vi "test_ReserveSessionForPinGroup_ReserveSuccessForPinsInGroup.vi"() -> (6 "pass":bool, 8 "result":string, 15 "error out":errorcluster)   [LabVIEW 2020]
uses:
  Runtime/MeasurementLink Pin Map Client/RPC Messages/ni_measurementlink_pinmap_v1_CreatePinMapFromXmlRequest.ctl
  Runtime/MeasurementLink Session Management Client/RPC Messages/ni_measurementlink_sessionmanagement_v1_ReserveSessionsRequest.ctl
  Runtime/MeasurementLink Session Management Client/RPC Messages/ni_measurementlink_PinMapContext.ctl
  Runtime/MeasurementLink Session Management Client/RPC Messages/ni_measurementlink_sessionmanagement_v1_ReserveAllRegisteredSessionsResponse.ctl
  3347d1b6-dca7-4e1a-9ca0-c9ec2f5aba95.vi
  ab61e54b-70f9-4719-86d2-c3025959eeb5.vi
  <vilib>/JDP Science/JSONtext/Variant to JSON Text.vi
  <vilib>/JDP Science/JSONtext/LVClass Serializer/JSONtext LVClass Serializer.lvclass
  Runtime/MeasurementLink Session Management Client/MeasurementLink Session Management Client.lvlib
  Runtime/MeasurementLink Pin Map Client/MeasurementLink Pin Map Client.lvlib
  Runtime/MeasurementLink Session Management Client/RPC Messages/ni_measurementlink_sessionmanagement_v1_ChannelMapping.ctl
  Runtime/MeasurementLink Session Management Client/RPC Messages/nidevice_grpc_Session.ctl
  Runtime/MeasurementLink Session Management Client/RPC Messages/ni_measurementlink_sessionmanagement_v1_SessionInformation.ctl
  Runtime/MeasurementLink Session Management Client/RPC Messages/ni_measurementlink_sessionmanagement_v1_MultiplexerSessionInformation.ctl
  Runtime/MeasurementLink Session Management Client/RPC Messages/ni_measurementlink_sessionmanagement_v1_ResolvedPinsOrRelays.ctl
  Runtime/MeasurementLink Session Management Client/RPC Messages/ni_measurementlink_sessionmanagement_v1_ReserveSessionsResponse_GroupMappingsEntry.ctl
  Runtime/MeasurementLink Session Management Client/RPC Messages/ni_measurementlink_sessionmanagement_v1_ReserveSessionsResponse.ctl
panel:
  # "Test assumes discovery service, pin map service, and session management service have already been started."
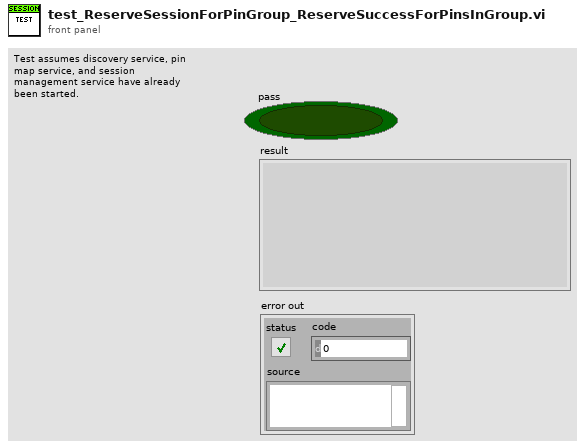
[diagram p1: front panel]
types:
  T1 = typedef "MeasurementLink Session Management Client.lvlib/ni_measurementlink_sessionmanagement_v1_ReserveSessionsResponse.ctl" = cluster{"sessions":T2[], "multiplexer_sessions":T5[], "group_mappings":T6[]}
  T2 = typedef "MeasurementLink Session Management Client.lvlib/ni_measurementlink_sessionmanagement_v1_SessionInformation.ctl" = cluster{"session":T3, "resource_name":string, "channel_list":string, "instrument_type_id":string, "session_exists":bool, "channel_mappings":T4[]}
  T3 = typedef "MeasurementLink Session Management Client.lvlib/nidevice_grpc_Session.ctl" = cluster{"name":string}
  T4 = typedef "MeasurementLink Session Management Client.lvlib/ni_measurementlink_sessionmanagement_v1_ChannelMapping.ctl" = cluster{"pin_or_relay_name":string, "site":i32, "channel":string, "multiplexer_resource_name":string, "multiplexer_route":string}
  T5 = typedef "MeasurementLink Session Management Client.lvlib/ni_measurementlink_sessionmanagement_v1_MultiplexerSessionInformation.ctl" = cluster{"session":T3, "resource_name":string, "multiplexer_type_id":string, "session_exists":bool}
  T6 = typedef "MeasurementLink Session Management Client.lvlib/ni_measurementlink_sessionmanagement_v1_ReserveSessionsResponse_GroupMappingsEntry.ctl" = cluster{"key":string, "value":T7}
  T7 = typedef "MeasurementLink Session Management Client.lvlib/ni_measurementlink_sessionmanagement_v1_ResolvedPinsOrRelays.ctl" = cluster{"pin_or_relay_names":string[]}
  T8 = typedef "MeasurementLink Session Management Client.lvlib/ni_measurementlink_sessionmanagement_v1_ReserveAllRegisteredSessionsResponse.ctl" = cluster{"sessions":T2[]}
  T9 = typedef "MeasurementLink Session Management Client.lvlib/ni_measurementlink_sessionmanagement_v1_ReserveSessionsRequest.ctl" = cluster{"pin_map_context":T10, "pin_or_relay_names":string[], "instrument_type_id":string, "timeout_in_milliseconds":i32}
  T10 = typedef "MeasurementLink Session Management Client.lvlib/ni_measurementlink_PinMapContext.ctl" = cluster{"pin_map_id":string, "sites":i32[]}
  T11 = typedef "MeasurementLink Pin Map Client.lvlib/ni_measurementlink_pinmap_v1_CreatePinMapFromXmlRequest.ctl" = cluster{"pin_map_id":string, "pin_map_xml":string}
  T12 = typedef "grpc-lvsupport-release.lvlib/grpcId.ctl" = u64
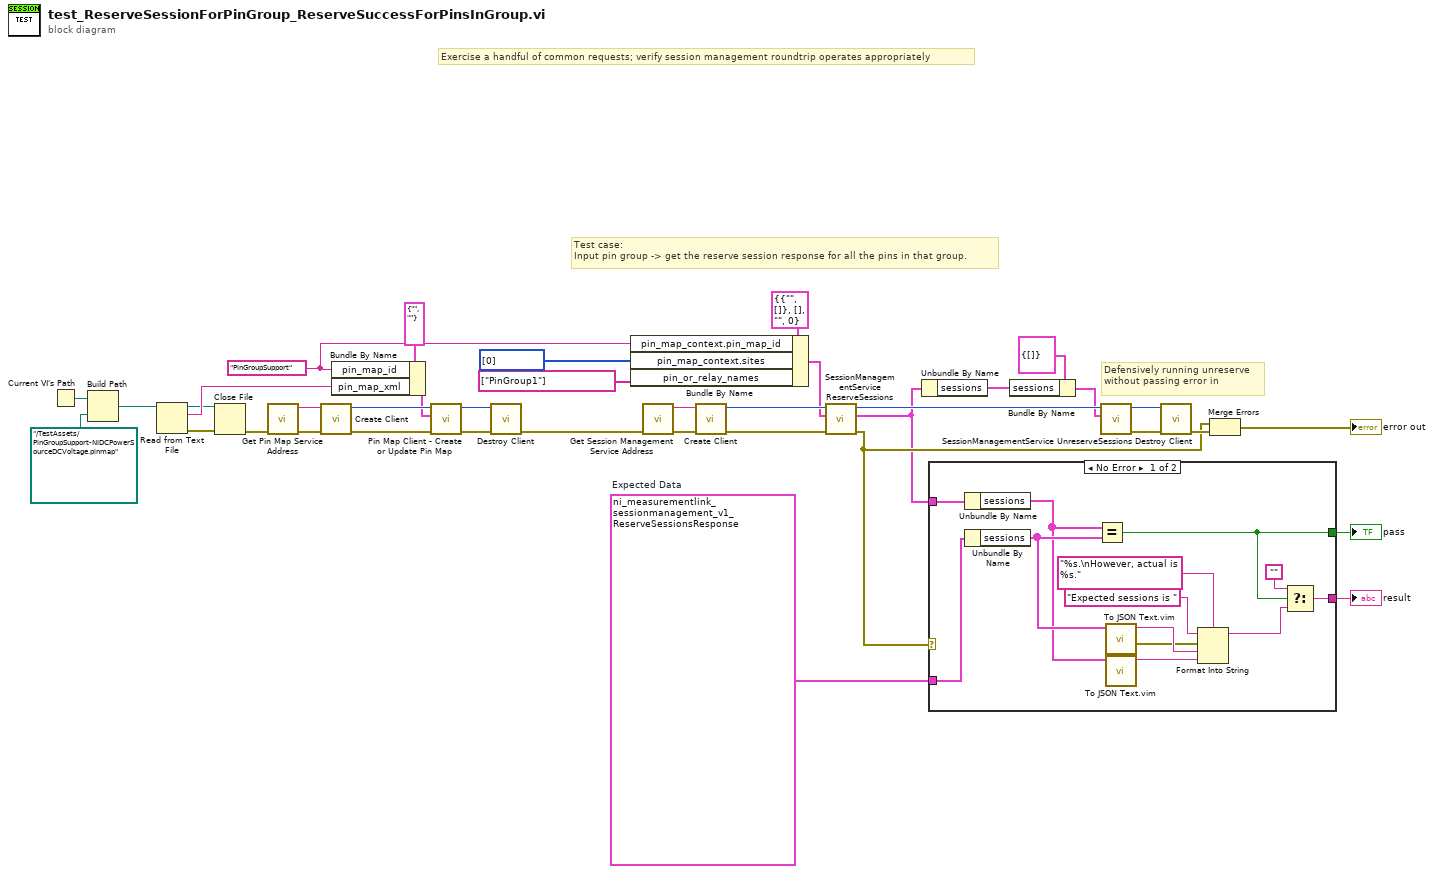
[diagram p0: block diagram]
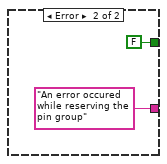
[diagram p2: hidden frame]
diagram:
  w1 = T1 {"sessions"=[{"session"={"name"="SMU_4140_A/0, SMU_4140_A/1, SMU_4140_A/2, SMU_4140_A/3"}, "resource_name"="SMU_4140_A/0, SMU_4140_A/1, SMU_4140_A/2, SMU_4140_A/3", "channel_list"="SMU_4140_A/0, SMU_4140_A/1", "instrument_type_id"="niDCPower", "session_exists"=FALSE, "channel_mappings"=[{"pin_or_relay_name"="Pin1", "site"=0, "channel"="SMU_4140_A/0", "multiplexer_resource_name"="", "multiplexer_route"=""}, {"pin_or_relay_name"="Pin2", "site"=0, "channel"="SMU_4140_A/1", "multiplexer_resource_name"="", "multiplexer_route"=""}]}], "multiplexer_sessions"=[], "group_mappings"=[{"key"="PinGroup1", "value"={"pin_or_relay_names"=["Pin1", "Pin2"]}}]}  # Expected Data
  w16 = "PinGroupSupport" ("pin_map_id")
  # "Test case:\nInput pin group -> get the reserve session response for all the pins in that group."
  # "Defensively running unreserve without passing error in"
  # "Exercise a handful of common requests; verify session management roundtrip operates appropriately"
  n1 = Current VI's Path() -> (path=w33:path)
  n2 = Build Path(base path=w33, name or relative path=path "../TestAssets/PinGroupSupport-NIDCPowerSourceDCVoltage.pinmap") -> (appended path=w31:path)
  n3 = Read from Text File(file (use dialog)=w31) -> (refnum out=w27:refnum<file>, text=w29:string, error out=w28:errorcluster)  [unwired: 3 in, 1 out]
  n4 = Close File(refnum=w27, error in=w28) -> (error out=w24:errorcluster)  [unwired: 1 out]
  n5 = call "Get Pin Map Service Address.vi"("error in (no error)"=w24) -> ("error out"=w25:errorcluster, "address"=w26:string)  [unwired: 9 in]
  n6 = call "Create Client.vi"("error in"=w25, "address"=w26) -> ("error out"=w34:errorcluster, "gRPC ID Out"=w23:T12)  [unwired: 8 in]
  n7 = Bundle By Name(cluster=T11 {"pin_map_id"="", "pin_map_xml"=""} ("Request Data"), "pin_map_id"=w16, "pin_map_xml"=w29) -> (w22:T11)
  n8 = call "Pin Map Client - Create or Update Pin Map.vi"("error in (no error)"=w34, "Request Data"=w22, "gRPC ID Out"=w23) -> ("error out"=w21:errorcluster, "gRPC ID out"=w20:T12)  [unwired: 6 in, 1 out]
  n9 = call "Destroy Client.vi"("error in"=w21, "gRPC ID"=w20) -> ("error out"=w19:errorcluster)  [unwired: 9 in]
  n10 = Bundle By Name(cluster=T9 {"pin_map_context"={"pin_map_id"="", "sites"=[]}, "pin_or_relay_names"=[], "instrument_type_id"="", "timeout_in_milliseconds"=0} ("Request Data"), "pin_map_context.pin_map_id"=w16, "pin_map_context.sites"=i32[] [0], "pin_or_relay_names"=string[] ["PinGroup1"]) -> (w11:T9)
  n11 = call "Get Session Management Service Address.vi"("error in (no error)"=w19) -> ("error out"=w38:errorcluster, "address"=w37:string)  [unwired: 9 in]
  n12 = call "Create Client.vi"("error in"=w38, "address"=w37) -> ("error out"=w36:errorcluster, "gRPC ID Out"=w35:T12)  [unwired: 8 in]
  n13 = call "SessionManagementService ReserveSessions.vi"("error in"=w36, "Request Data"=w11, "gRPC ID"=w35) -> ("error out"=w6:errorcluster, "Response Data"=w2:T1, "gRPC ID out"=w12:T12)  [unwired: 6 in]
  n14 = Unbundle By Name(w2) -> ("sessions"=w4:T2[])
  n15 = case shown="No Error" w6 {
    tunnel: [w49 FALSE] -> w10
    tunnel: [w48 "An error occured while reserving the pin group" ("String")] -> w9
    tunnel: w2 -> [w50 _]
    tunnel: w1 -> [w51 _]
    frame No Error {
      n16 = Unbundle By Name(w50) -> ("sessions"=w41:T2[])
      n17 = Unbundle By Name(w51) -> ("sessions"=w44:T2[])
      n18 = Equal?(x=w41, y=w44) -> (x = y?=w49:bool)
      n19 = call "To JSON Text.vim"("Anything"=w44) -> ("error out"=w42:errorcluster, "<JSON>"=w43:string)  [unwired: 9 in]
      n20 = call "To JSON Text.vim"("Anything"=w41) -> ("<JSON>"=w40:string)  [unwired: 9 in, 1 out]
      n21 = Format Into String(format string="%s.\nHowever, actual is %s.", initial string="Expected sessions is ", error in=w42, w43, w40) -> (resulting string=w39:string)  [unwired: 1 out]
      n22 = Select(t="", s=w49, f=w39) -> (s? t:f=w48:string)
    }
    frame Error {
    }
  }
  "pass" <- w10
  "result" <- w9
  n23 = Bundle By Name(cluster=T8 {"sessions"=[]} ("response data 2"), "sessions"=w4) -> (w3:T8)
  n24 = call "SessionManagementService UnreserveSessions.vi"("Request Data"=w3, "gRPC ID"=w12) -> ("error out"=w13:errorcluster, "gRPC ID out"=w18:T12)  [unwired: 7 in, 1 out]
  n25 = call "Destroy Client.vi"("error in"=w13, "gRPC ID"=w18) -> ("error out"=w8:errorcluster)  [unwired: 9 in]
  n26 = Merge Errors(w6, w8) -> (→"error out":errorcluster)
